vi "timerfd test.vi"() -> ()   [LabVIEW 2016]
uses:
  Source/C/Controls/epoll operations.ctl
  Source/C/Controls/epoll events.ctl
  Source/C/SubVIs/OR flags U32.vi
  <vilib>/NI/NI Linux RT Utilities/VIs/Public/Convert Types/convert timespec 64 to timespec 32.vi
  <vilib>/NI/NI Linux RT Utilities/VIs/Public/Convert Types/convert timespec 32 to timespec 64.vi
  <vilib>/NI/NI Linux RT Errno/VIs/Public/Get Errno Value for Calling Thread.vi
  Source/C/SubVIs/error handler.vi
  Source/C/Linux RT IPC.C.lvlib
panel:
  out "timed out":bool
  out "number of ready fds":i32
  out "error out":errorcluster
  out "iterations":i32
  in  "stop":bool
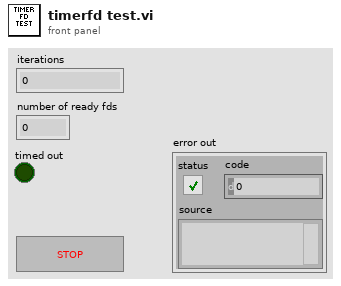
[diagram p1: front panel]
types:
  T1 = typedef "Linux RT IPC.C.lvlib/epoll events.ctl" = u32
  T2 = typedef "Linux RT IPC.C.lvlib/epoll operations.ctl" = u32
  T3 = cluster{"it_interval":cluster{"sec":u64, "nsec":u64}, "it_value":cluster{"sec":u64, "nsec":u64}}
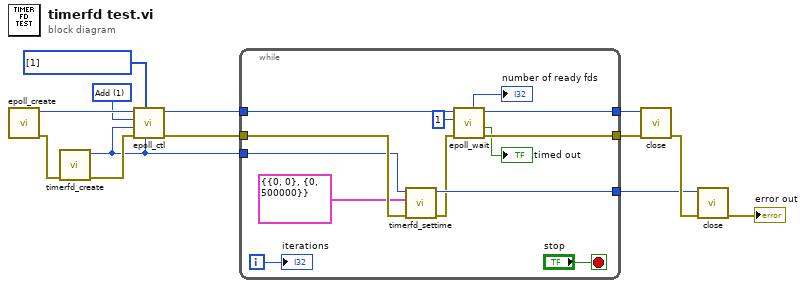
[diagram p0: block diagram]
diagram:
  w10 = T1[] [1] items=["EPOLLIN"=1, "EPOLLPRI"=2, "EPOLLOUT"=4, "EPOLLERR"=8, "EPOLLHUP"=16, "EPOLLRDNORM"=64, "EPOLLRDBAND"=128, "EPOLLWRNORM"=256, "EPOLLWRBAND"=512, "EPOLLMSG"=1024, "EPOLLRDHUP"=8192, "EPOLLWAKEUP"=536870912, "EPOLLONESHOT"=1073741824, "EPOLLET"=2147483648] ("epoll events (default: none)")
  w11 = T2 1 items=["Add"=1, "Delete"=2, "Modify"=3] ("operation")
  n1 = call "epoll_create.vi"() -> ("error out"=w13:errorcluster, "epfd"=w12:i32)  [unwired: 10 in]
  n2 = call "timerfd_create.vi"("error in (no error)"=w13) -> ("error out"=w9:errorcluster, "timer fd"=w5:i32)  [unwired: 9 in]
  n3 = call "epoll_ctl.vi"("epoll data"=w5, "epoll events (default: none)"=w10, "error in (no error)"=w9, "target fd"=w5, "operation"=w11, "epfd in"=w12) -> ("error out"=w6:errorcluster, "epfd out"=w8:i32)  [unwired: 4 in]
  n4 = while {
    tunnel: w8 -> [w24]
    tunnel: [w23] -> w7
    tunnel: w6 -> [w26]
    tunnel: w5 -> [w22]
    tunnel: [w21] -> w2
    tunnel: [w16] -> w4
    i -> [w19]
    stop <- "stop" stop-if-true
    n5 = call "timerfd_settime.vi"("error in (no error)"=w26, "new value"=T3 {"it_interval"={"sec"=0, "nsec"=0}, "it_value"={"sec"=0, "nsec"=500000}}, "fd in"=w22) -> ("error out"=w18:errorcluster, "fd out"=w21:i32)  [unwired: 6 in, 1 out]
    n6 = call "epoll_wait.vi"("error in (no error)"=w18, "max events"=u32 1, "epfd in"=w24) -> ("error out"=w16:errorcluster, "timed out"=→"timed out":bool, "epfd out"=w23:i32, "number of ready fds"=→"number of ready fds":i32)  [unwired: 4 in, 1 out]
    "iterations" <- w19
  }
  n7 = call "close.vi"("error in (no error)"=w4, "file descriptor in"=w7) -> ("error out"=w3:errorcluster)  [unwired: 9 in]
  n8 = call "close.vi"("error in (no error)"=w3, "file descriptor in"=w2) -> ("error out"=→"error out":errorcluster)  [unwired: 9 in]
